vi "FA_MultiReadXML.vi"(6 "Error In":errorcluster, 8 "Special Type Array":T1[](array[typedef])) -> (0 "Error Out":errorcluster, 2 "XML String Array":string[](array[string]))   [LabVIEW 2014, in "FA_LocalStore.lvlib"]
doc: "Returnsan array of XML from LocalStore for an array of Special Type."
uses:
  FA_LocalStore.lvlib
  FA_LSSpecialTypes.ctl
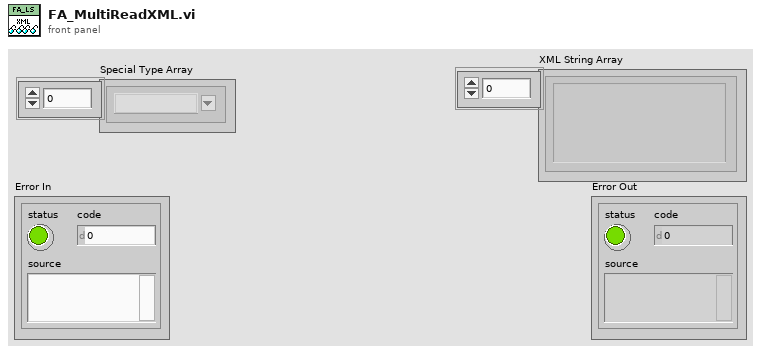
[diagram p1: front panel]
types:
  T1 = typedef "FA_LocalStore.lvlib/FA_LSSpecialTypes.ctl" = string
  T2 = typedef "FA_LocalStore.lvlib/FA_LSRef.ctl" = cluster{"eTag INI Refnum":T3, "XML Refnum Array":refnum<file>[]}
  T3 = typedef "NI_LVConfig.lvlib/Config Data RefNum.ctl" = refnum<k1>
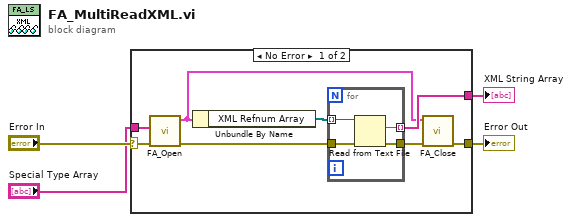
[diagram p0: block diagram]
diagram:
  n1 = case shown="No Error" "Error In" {
    selector: "Error In" -> [w11 w17]
    tunnel: [w8 w17] -> w4
    tunnel: "Special Type Array" -> [w6 _]
    tunnel: [w12 _] -> w1
    frame No Error {
      n2 = call "FA_Open.vi"("Error In"=w11, "Special Types Array"=w6) -> ("Error Out"=w7:errorcluster, "FA_LS Ref"=w10:T2)  [unwired: 8 in]
      n3 = Unbundle By Name(w10) -> ("XML Refnum Array"=w5:refnum<file>[])
      n4 = for {
        tunnel: [w16] -> w12 mode=indexing
        tunnel: [w15] -> w9
        tunnel: w7 -> [w14]
        tunnel: w5 -> [w13] mode=indexing
        n5 = Read from Text File(file (use dialog)=w13, error in=w14) -> (text=w16:string, error out=w15:errorcluster)  [unwired: 2 in, 2 out]
      }
      n6 = call "FA_Close.vi"("Error In"=w9, "FA_LS Ref"=w10) -> ("Error Out"=w8:errorcluster)  [unwired: 9 in]
    }
    frame Error {
    }
  }
  "Error Out" <- w4
  "XML String Array" <- w1
